vi "Pickup Area.vi"(1 "Path Positions":T1(array[cluster]), 2 "Min Pos Bound":cluster{"x setpoint":dbl, "y setpoint":dbl}, 3 "Max Pos Bound":cluster{"x setpoint":dbl, "y setpoint":dbl}) -> (0 "Path Positions":T1(array[cluster]))   [LabVIEW 2025]
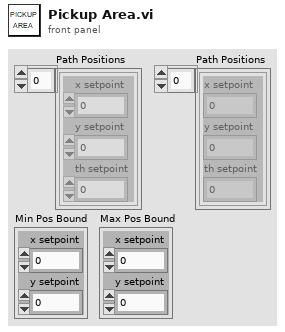
[diagram p1: front panel]
types:
  T1 = cluster{"x setpoint":dbl, "y setpoint":dbl, "th setpoint":dbl}[]
  T2 = cluster{"x setpoint":dbl, "y setpoint":dbl, "th setpoint":dbl}
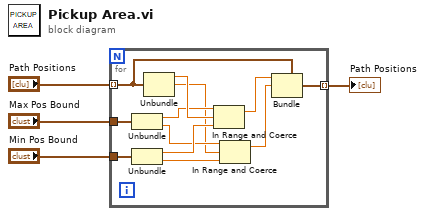
[diagram p0: block diagram]
diagram:
  n1 = for {
    tunnel: "Path Positions" -> [w16] mode=indexing
    tunnel: [w15] -> w3 mode=indexing
    tunnel: "Max Pos Bound" -> [w14]
    tunnel: "Min Pos Bound" -> [w13]
    n2 = Unbundle(w14) -> ("x setpoint"=w11:dbl, "y setpoint"=w7:dbl)
    n3 = Unbundle(w13) -> ("x setpoint"=w10:dbl, "y setpoint"=w8:dbl)
    n4 = Unbundle(w16) -> ("x setpoint"=w12:dbl, "y setpoint"=w5:dbl)  [unwired: 1 out]
    n5 = In Range and Coerce(upper limit=w11, x=w12, lower limit=w10) -> (coerced(x)=w9:dbl)  [unwired: 1 out]
    n6 = In Range and Coerce(upper limit=w7, x=w5, lower limit=w8) -> (coerced(x)=w6:dbl)  [unwired: 1 out]
    n7 = Bundle(cluster=w16, "x setpoint"=w9, "y setpoint"=w6) -> (w15:T2)  [unwired: 1 in]
  }
  "Path Positions" <- w3
